vi "CHD_DRIVE_GET_MAX.vi"() -> (3 "Max Wheel Vel (Meter/Sec)":dbl)   [LabVIEW 2019]
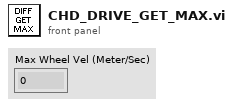
[diagram p1: front panel]
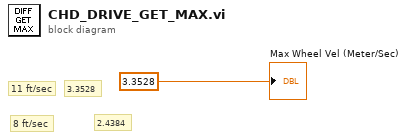
[diagram p0: block diagram]
diagram:
  # "11 ft/sec"
  # "2.4384"
  # "3.3528"
  # "8 ft/sec"
  "Max Wheel Vel (Meter/Sec)" <- 3.3528
